vi "NIDCPower_channel_ganging - confgure sequence.vi"(6 "output function":T1=1007 caption="Output Function" items=["DC Voltage"=1006, "DC Current"=1007, "Pulse Voltage"=1049, "Pulse Current"=1050], 8 "error in (no error)":errorcluster, 9 "Source Delays":dbl[](array[numeric]), 10 "Values":dbl[](array[numeric]), 11 "Ganged Session In":T2) -> (0 "error out":errorcluster, 3 "Ganged Session Out":T2)   [LabVIEW 2021]
uses:
  ctl/NIDCPower_channel_ganging - ctl - ganged config.ctl
  ctl/NIDCPower_channel_ganging - ctl - channel mode.ctl
  ctl/NIDCPower_channel_ganging - ctl - ganged session.ctl
  <instrlib>/niDCPower/nidcpower.llb/niDCPower Output Function.ctl
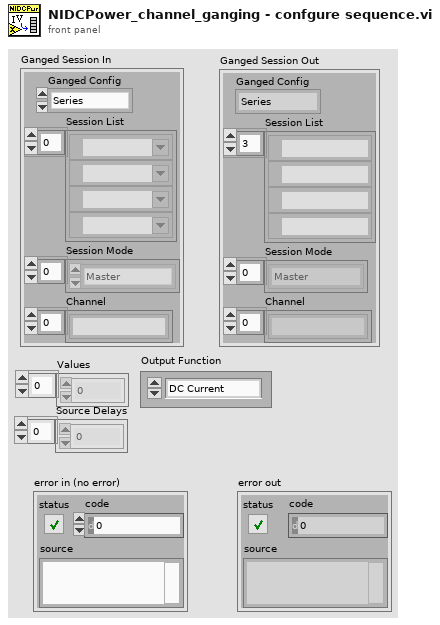
[diagram p1: front panel]
types:
  T1 = typedef "niDCPower Output Function.ctl" = i32
  T2 = typedef "NIDCPower_channel_ganging - ctl - ganged session.ctl" = cluster{"Ganged Config":T3, "Session List":refnum<k15>[], "Session Mode":T4[], "Channel":string[]}
  T3 = typedef "NIDCPower_channel_ganging - ctl - ganged config.ctl" = enum16{"Series", "Parallel", "Manual"}
  T4 = typedef "NIDCPower_channel_ganging - ctl - channel mode.ctl" = enum16{"Master", "Slave", "Slave - Inverted"}
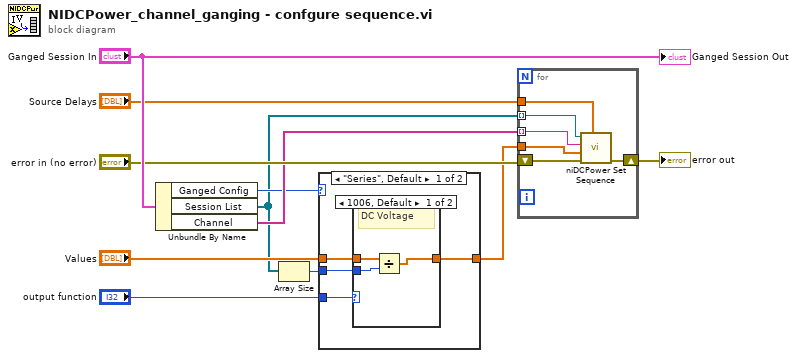
[diagram p0: block diagram]
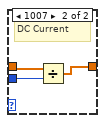
[diagram p4: hidden frame]
diagram:
  n1 = Unbundle By Name("Ganged Session In") -> ("Ganged Config"=w6:T3, "Session List"=w2:refnum<k15>[], "Channel"=w7:string[])
  n2 = Array Size(array=w2) -> (size(s)=w1:i32)
  n3 = case shown="\"Series\", Default" w6 {
    tunnel: "Values" -> [w15 w23]
    tunnel: "output function" -> [w12 w22]
    tunnel: [w14 w21] -> w3
    tunnel: w1 -> [w13 w20]
    frame "Series", Default {
      n4 = case shown="1006, Default" w12 {
        tunnel: w15 -> [w18 w19]
        tunnel: [w17 w19] -> w14
        tunnel: w13 -> [w16 _]
        frame 1006, Default {
          # "DC Voltage"
          n5 = Divide(x=w18, y=w16) -> (x/y=w17:dbl[])
        }
        frame 1007 {
          # "DC Current"
        }
      }
    }
    frame "Parallel" {
      n6 = case shown="1006, Default" w22 {
        tunnel: w23 -> [w24 w27]
        tunnel: [w24 w25] -> w21
        tunnel: w20 -> [_ w26]
        frame 1006, Default {
          # "DC Voltage"
        }
        frame 1007 {
          # "DC Current"
          n7 = Divide(x=w27, y=w26) -> (x/y=w25:dbl[])
        }
      }
    }
  }
  n8 = for {
    tunnel: w2 -> [w33] mode=indexing
    tunnel: w3 -> [w32]
    shift-right: [w31] -> w9
    shift-left: "error in (no error)" -> [w30]
    tunnel: "Source Delays" -> [w29]
    tunnel: w7 -> [w28] mode=indexing
    n9 = call <instrlib>:"niDCPower Set Sequence.vi"("source delays"=w29, "error in (no error)"=w30, "values"=w32, "channel name"=w28, "instrument handle"=w33) -> ("error out"=w31:errorcluster)  [unwired: 6 out]
  }
  "error out" <- w9
  "Ganged Session Out" <- "Ganged Session In"
